vi "validate data.vi"(11 "Template in":refnum<class "Template.lvclass">) -> (0 "error out":errorcluster, 2 "Data valid?":bool, 3 "Template out":refnum<class "Template.lvclass">)   [LabVIEW 2020, in "Template.lvlib" / "Template.lvclass"]
uses:
  Template.lvclass
  Template.lvclass/Template.ctl
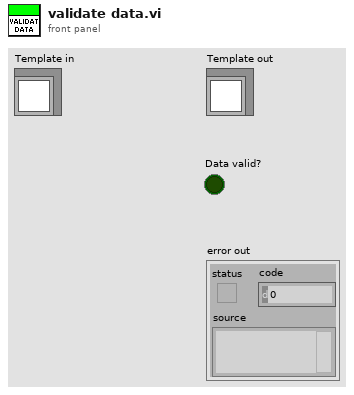
[diagram p1: front panel]
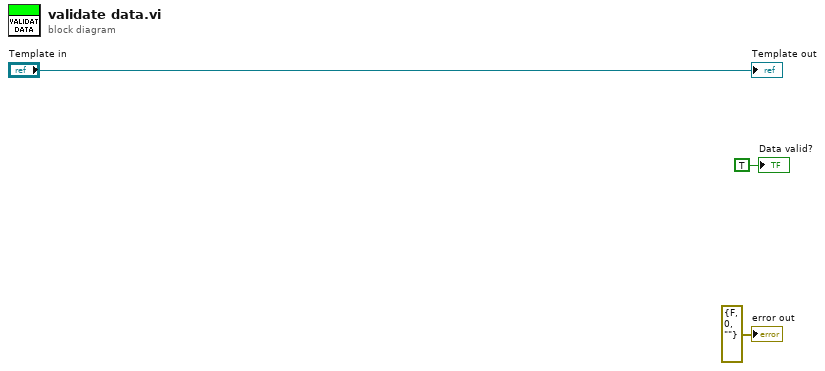
[diagram p0: block diagram]
diagram:
  "error out" <- errorcluster {"status"=FALSE, "code"=0, "source"=""} ("error out")
  "Template out" <- "Template in"
  "Data valid?" <- TRUE ("Data valid?")
